vi "SCD - Run Cookbook.vi"(5 "demo":bool, 6 "Timestamp at Start":timestamp=timestamp(3498061709.3036537 s since 1904-01-01), 7 "Neo Info":T10={"Handle"=102, "Pixel Encoding"="Mono16", "AOI Width"=2560, "AOI Height"=2160, "AOI Stride"=5136, "Image Bytes"=11098896, "Image Pixels"=5529600, "Row Readout Time"=9.371428571428572e-06, "Frame Readout Time"=0.010121142857142858, "Interframe Time"=8.434285714285715e-05, "Semaphore"=refnum, "SerialNumber"="SCC-02209", "Camera Model"="DC-152Q-C00-FI", "Controller ID"="3", "Firmware Version"="13.8.26.122", "Shutter"="Global", "Binning"=0, "Time at Synch"=timestamp(3029526000.379448 s since 1904-01-01), "Idx"=0} {"Time at Synch" format="%<%H:%M:%S>T"; "Interframe Time" format="%#_3g"; "Frame Readout Time" format="%_3g"; "Row Readout Time" format="%_3g"}, 8 "Error in":errorcluster, 9 "FITS Header In":T1={"Wavelength (nm)"=530.15, "Exposure (s)"=0.05, "Tuning Delay (ms)"=1000.0, "Beam Type (-1/1)"=1.0, "Tuning Voltages"=[1.111, 2.222, 3.333, 4.444], "Observer"="observer", "Light Shapping Diffuser"=enum."In Beam", "Comment"="", "Data Type"=9, "Mod Cycles"=0, "SCD Calibration Optics"=enum."1 - Polarizer @0, I+Q", "SCD Emission Line Filter"=enum."1-557.6nm", "Cookbook"="", "COMP-S Calibration Wheel"=enum."Dark", "COMP-S Andover Filter Wheel"=enum."530.3nm/HWB 0.34nm (Fe XIV)", "FOV Rotation (deg)"=66.0, "Objective Lens Position (mm)"=0.0, "Occulter size"=0.0, "Time End"=timestamp(3382374145.421875 s since 1904-01-01), "Acc Exposure (s)"=0.0, "Time Stamp Array"=[], "Camera Serial Number"=[], "Camera Temp"=[], "Camera PI (mm)"=[0.0, 0.0, 0.0], "Time Start"=timestamp(3382374145.421875 s since 1904-01-01), "Peripherals"={"ILX controler"=FALSE, "Zone temperatures"=FALSE, "Andor"=FALSE, "Andor 2"=FALSE, "PI Stages"=FALSE, "AISAS mechanisms"=FALSE, "AISAS Mech.lvclass"=refnum, "Zone temp ref"=variant, "FWs"=FALSE}, "FITS paths"=[path " ", path " ", path " ", path " "], "Cameras"=enum."Andor", "load preset cbk"=FALSE, "periodic check count"=0} {"Camera PI (mm)" format="%_3g"; "Acc Exposure (s)" format="%^.3g"; "Occulter size" format="%.2f"; "Objective Lens Position (mm)" min=70.0 max=152.0 format="%.2f"; "FOV Rotation (deg)" format="%.1f"; "Data Type" items=["LIVE", "DARK", "FLAT", "CALI", "OBSE", "ABSO", "AURE", "TARG", "OBJE", "HOLE", "OREX", "THRO", "CHIP"]; "Exposure (s)" format="%^.3g"; "Wavelength (nm)" format="%_6g"}, 10 "FPS":dbl=20.0 format="%0.2p", 11 "Cookbook":T12(array[cluster])=[{"Data Type"=enum."SET EXPOSURE", "Arg 1"=0.1, "Arg 2"=999.0, "Arg 3"=path "C:/SCD Cookbooks/exposure-100ms.rcp", "Comments"=""}, {"Data Type"=enum."ACQUIRE DATA", "Arg 1"=1.0, "Arg 2"=1.0, "Arg 3"=path "C:/SCD Cookbooks/aaa.rcp", "Comments"=""}]) -> (0 "Error out":errorcluster={"status"=FALSE, "code"=5000, "source"="AT Clear All Buffers A.vi\n\nSUCCESS"}, 1 "Headers Out":T1[](array[typedef]) {"Camera PI (mm)" format="%_3g"; "Acc Exposure (s)" format="%^.3g"; "Occulter size" format="%.2f"; "Objective Lens Position (mm)" min=70.0 max=152.0 format="%.2f"; "FOV Rotation (deg)" format="%.1f"; "Data Type" items=["LIVE", "DARK", "FLAT", "CALI", "OBSE", "ABSO", "AURE", "TARG", "OBJE", "HOLE", "OREX", "THRO", "CHIP"]; "Exposure (s)" format="%^.3g"; "Wavelength (nm)" format="%_6g"}, 2 "FITS Path Out":path, 3 "Result":string)   [LabVIEW 2014]
doc: "Use this template to build a VI to use as a subVI."
uses:
  AISAS/Controls/Diffuser.ctl
  <vilib>/Utility/file.llb/Read From Spreadsheet File (DBL).vi
  Controls/SCD - Calibration Optics Filter Wheel.ctl
  Controls/SCD - FITS Cluster.ctl
  Camera/Andor Neo Info.ctl
  Controls/SCD - EDT - Emission Line Filter Wheel.ctl
  Controls/CoMP-S Controls/Polarization Optics Filter Wheel.ctl
  Controls/CoMP-S Controls/Emission Line Filter Wheel.ctl
  AISAS/Controls/focus.ctl
  AISAS/Mech/AISAS Mech.lvclass
  Controls/peripherals.ctl
  Controls/Cameras select.ctl
panel:
  in  "Stop Cookbook":bool
  out "Recipe Being Processed":string
  out "Most Recent Image Accumulation (Modulation State A)":u32[][](graph)
  out "Changes 0 or 1 to true/false for absolute or relative control":bool[](array[boolean])
  out "Updated Header":T1={"Wavelength (nm)"=530.15, "Exposure (s)"=0.05, "Tuning Delay (ms)"=1000.0, "Beam Type (-1/1)"=1.0, "Tuning Voltages"=[1.111, 2.222, 3.333, 4.444], "Observer"="observer", "Light Shapping Diffuser"=enum."In Beam", "Comment"="", "Data Type"=9, "Mod Cycles"=0, "SCD Calibration Optics"=enum."1 - Polarizer @0, I+Q", "SCD Emission Line Filter"=enum."1-557.6nm", "Cookbook"="", "COMP-S Calibration Wheel"=enum."Dark", "COMP-S Andover Filter Wheel"=enum."530.3nm/HWB 0.34nm (Fe XIV)", "FOV Rotation (deg)"=66.0, "Objective Lens Position (mm)"=0.0, "Occulter size"=0.0, "Time End"=timestamp(3382374145.421875 s since 1904-01-01), "Acc Exposure (s)"=0.0, "Time Stamp Array"=[], "Camera Serial Number"=[], "Camera Temp"=[], "Camera PI (mm)"=[0.0, 0.0, 0.0], "Time Start"=timestamp(3382374145.421875 s since 1904-01-01), "Peripherals"={"ILX controler"=FALSE, "Zone temperatures"=FALSE, "Andor"=FALSE, "Andor 2"=FALSE, "PI Stages"=FALSE, "AISAS mechanisms"=FALSE, "AISAS Mech.lvclass"=refnum, "Zone temp ref"=variant, "FWs"=FALSE}, "FITS paths"=[path " ", path " ", path " ", path " "], "Cameras"=enum."Andor", "load preset cbk"=FALSE, "periodic check count"=0} {"Camera PI (mm)" format="%_3g"; "Acc Exposure (s)" format="%^.3g"; "Occulter size" format="%.2f"; "Objective Lens Position (mm)" min=70.0 max=152.0 format="%.2f"; "FOV Rotation (deg)" format="%.1f"; "Data Type" items=["LIVE", "DARK", "FLAT", "CALI", "OBSE", "ABSO", "AURE", "TARG", "OBJE", "HOLE", "OREX", "THRO", "CHIP"]; "Exposure (s)" format="%^.3g"; "Wavelength (nm)" format="%_6g"}
  out "LCVR Voltages":dbl[][](array[numeric])
  out "Total Recipes":i32=2
  out "Recipe Step":i32=1
  out "Mod Cycles":u16=1
  out "Exposure (s)":sgl=0.1
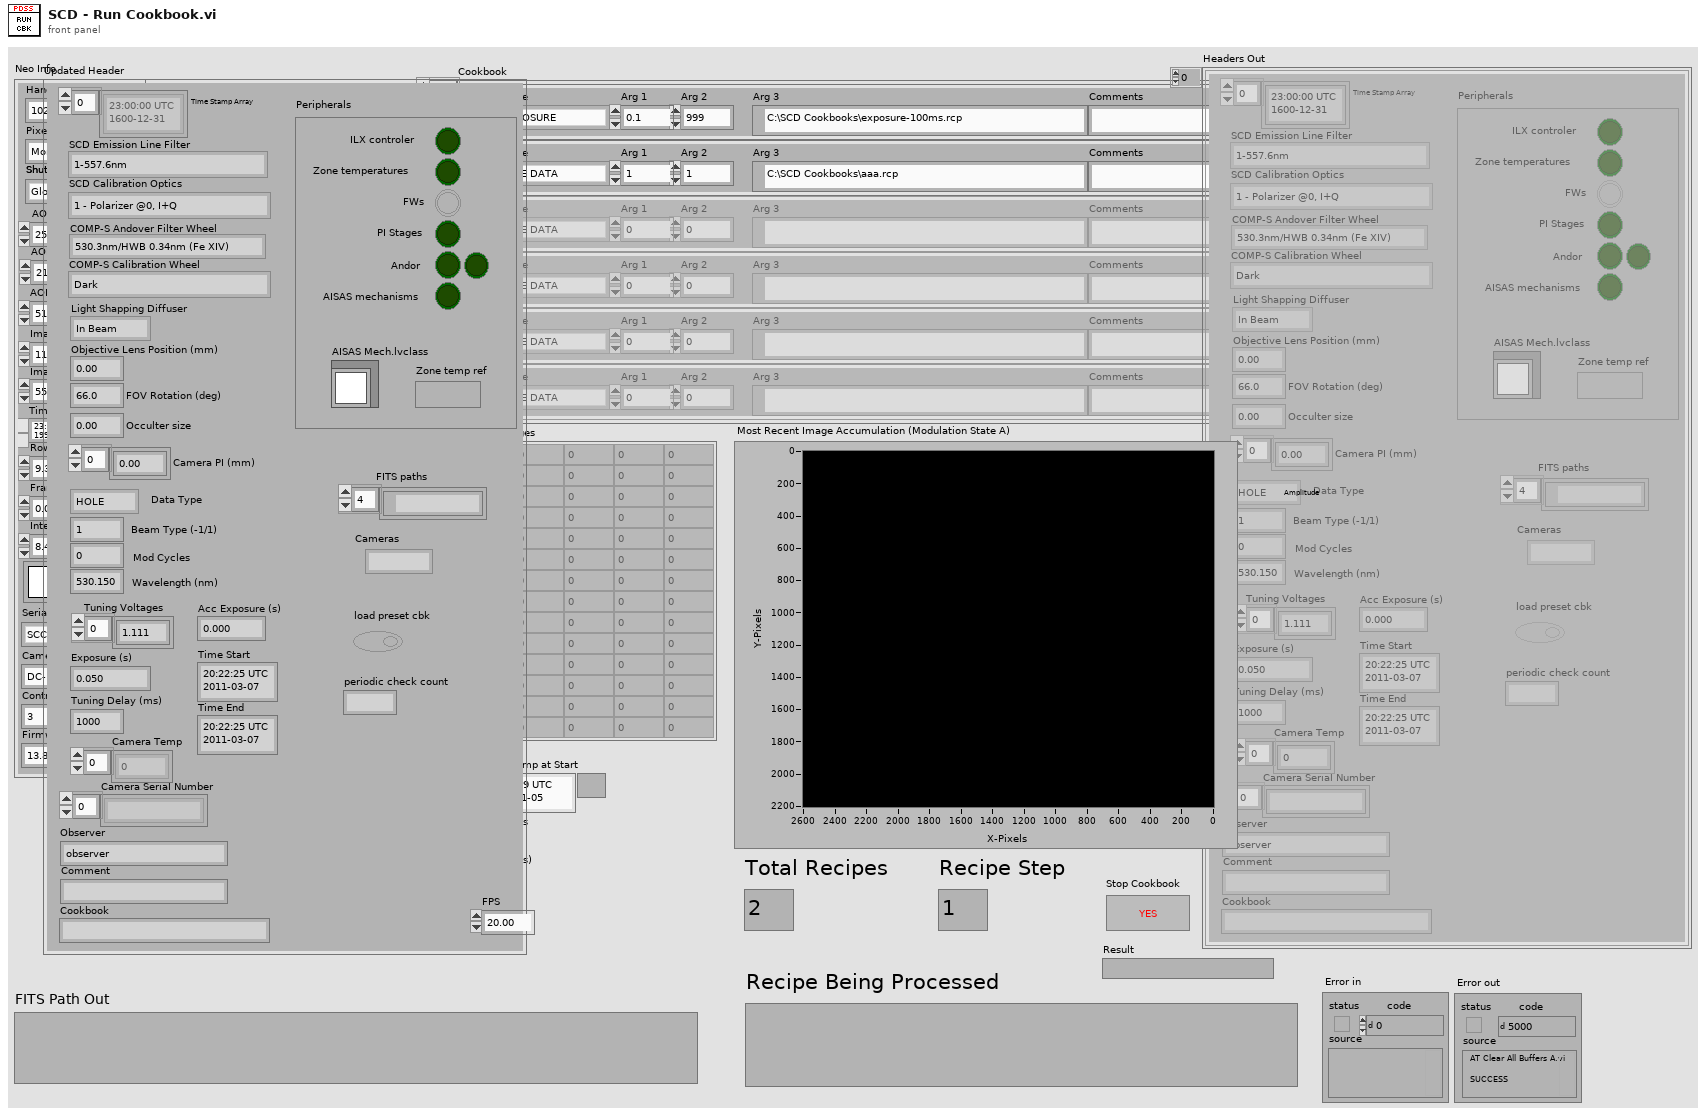
[diagram p1: front panel]
types:
  T1 = typedef "SCD - FITS Cluster.ctl" = cluster{"Wavelength (nm)":dbl, "Exposure (s)":dbl, "Tuning Delay (ms)":dbl, "Beam Type (-1/1)":dbl, "Tuning Voltages":dbl[], "Observer":string, "Light Shapping Diffuser":T2, "Comment":string, "Data Type":u16, "Mod Cycles":u16, "SCD Calibration Optics":T3, "SCD Emission Line Filter":T4, "Cookbook":string, "COMP-S Calibration Wheel":T5, "COMP-S Andover Filter Wheel":T6, "FOV Rotation (deg)":dbl, "Objective Lens Position (mm)":T7, "Occulter size":dbl, "Time End":timestamp, "Acc Exposure (s)":dbl, "Time Stamp Array":timestamp[], "Camera Serial Number":string[], "Camera Temp":dbl[], "Camera PI (mm)":dbl[], "Time Start":timestamp, "Peripherals":T8, "FITS paths":path[], "Cameras":T9, "load preset cbk":bool, "periodic check count":i32}
  T2 = typedef "Diffuser.ctl" = enum16{"Out of Beam", "In Beam"}
  T3 = typedef "SCD - Calibration Optics Filter Wheel.ctl" = enum16{"1 - Polarizer @0, I+Q", "2 - Polarizer @90, I-Q", "3 - Polarizer @45, I+U", "4 - Polarizer @135, I-U", "5 - Polarizer @0, Retarder @45, I+V", "6 - Polarizer @0, Retarder @135, I-V", "7 - Dark", "8 - Clear", "9 - N/A"}
  T4 = typedef "SCD - EDT - Emission Line Filter Wheel.ctl" = enum16{"1-557.6nm", "2-587.6nm", "3-589.6nm", "4-630.2nm", "5-656.4nm", "6-849.8nm", "7-854.2nm", "8-866.2nm", "9-1083.0nm"}
  T5 = typedef "Polarization Optics Filter Wheel.ctl" = enum16{"Dark", "Clear", "Exchange Lens", "Polarizer @0, I+Q", "Polarizer @90, I-Q", "Polarizer @45, I+U", "Polarizer @135, I-U", "Polarizer @0, Retarder @45, I+V", "Polarizer @0, Retarder @135, I-V"}
  T6 = typedef "Emission Line Filter Wheel.ctl" = enum16{"530.3nm/HWB 0.34nm (Fe XIV)", "587.6nm/HBW 0.44nm (He I D3)", "637.5nm/HBW 0.53nm (Fe X)", "656.3nm/HBW 0.57nm (H-Alpha)", "789.2nm/HBW 0.85nm (Fe XI)", "854.2nm/HBW 1.01nm (Ca I)", "1074.7nm/HBW 2.34nm (Fe XIII)", "1079.8nm/HBW 1.64nm (Fe XIII)", "1083.0nm/HBW 1.66nm (He I)"}
  T7 = typedef "focus.ctl" = dbl
  T8 = typedef "peripherals.ctl" = cluster{"ILX controler":bool, "Zone temperatures":bool, "Andor":bool, "Andor 2":bool, "PI Stages":bool, "AISAS mechanisms":bool, "AISAS Mech.lvclass":refnum<class "AISAS Mech.lvclass">, "Zone temp ref":variant, "FWs":bool}
  T9 = typedef "Cameras select.ctl" = enum16{"Andor", "GDR"}
  T10 = typedef "Andor Neo Info.ctl" = cluster{"Handle":i32, "Pixel Encoding":string, "AOI Width":i64, "AOI Height":i64, "AOI Stride":i64, "Image Bytes":i64, "Image Pixels":i64, "Row Readout Time":dbl, "Frame Readout Time":dbl, "Interframe Time":dbl, "Semaphore":T11, "SerialNumber":string, "Camera Model":string, "Controller ID":string, "Firmware Version":string, "Shutter":string, "Binning":u8, "Time at Synch":timestamp, "Idx":i32}
  T11 = typedef "Semaphore RefNum" = refnum<k1>
  T12 = cluster{"Data Type":enum32{"ACQUIRE DATA", "SET DIFFUSER", "CAL-FW", "WAVELENGTH-FW", "INSTR. ROTATION", "MOVE-ABS", "DATATYPE", "SET EXPOSURE", "CBK COMMENTS", "MOVE-REL"}, "Arg 1":sgl, "Arg 2":sgl, "Arg 3":path, "Comments":string}[]
  T13 = enum16{"Emission Line Filters", "Calibration Polarizers"}
  T14 = enum32{"ACQUIRE DATA", "SET DIFFUSER", "CAL-FW", "WAVELENGTH-FW", "INSTR. ROTATION", "MOVE-ABS", "DATATYPE", "SET EXPOSURE", "CBK COMMENTS", "MOVE-REL"}
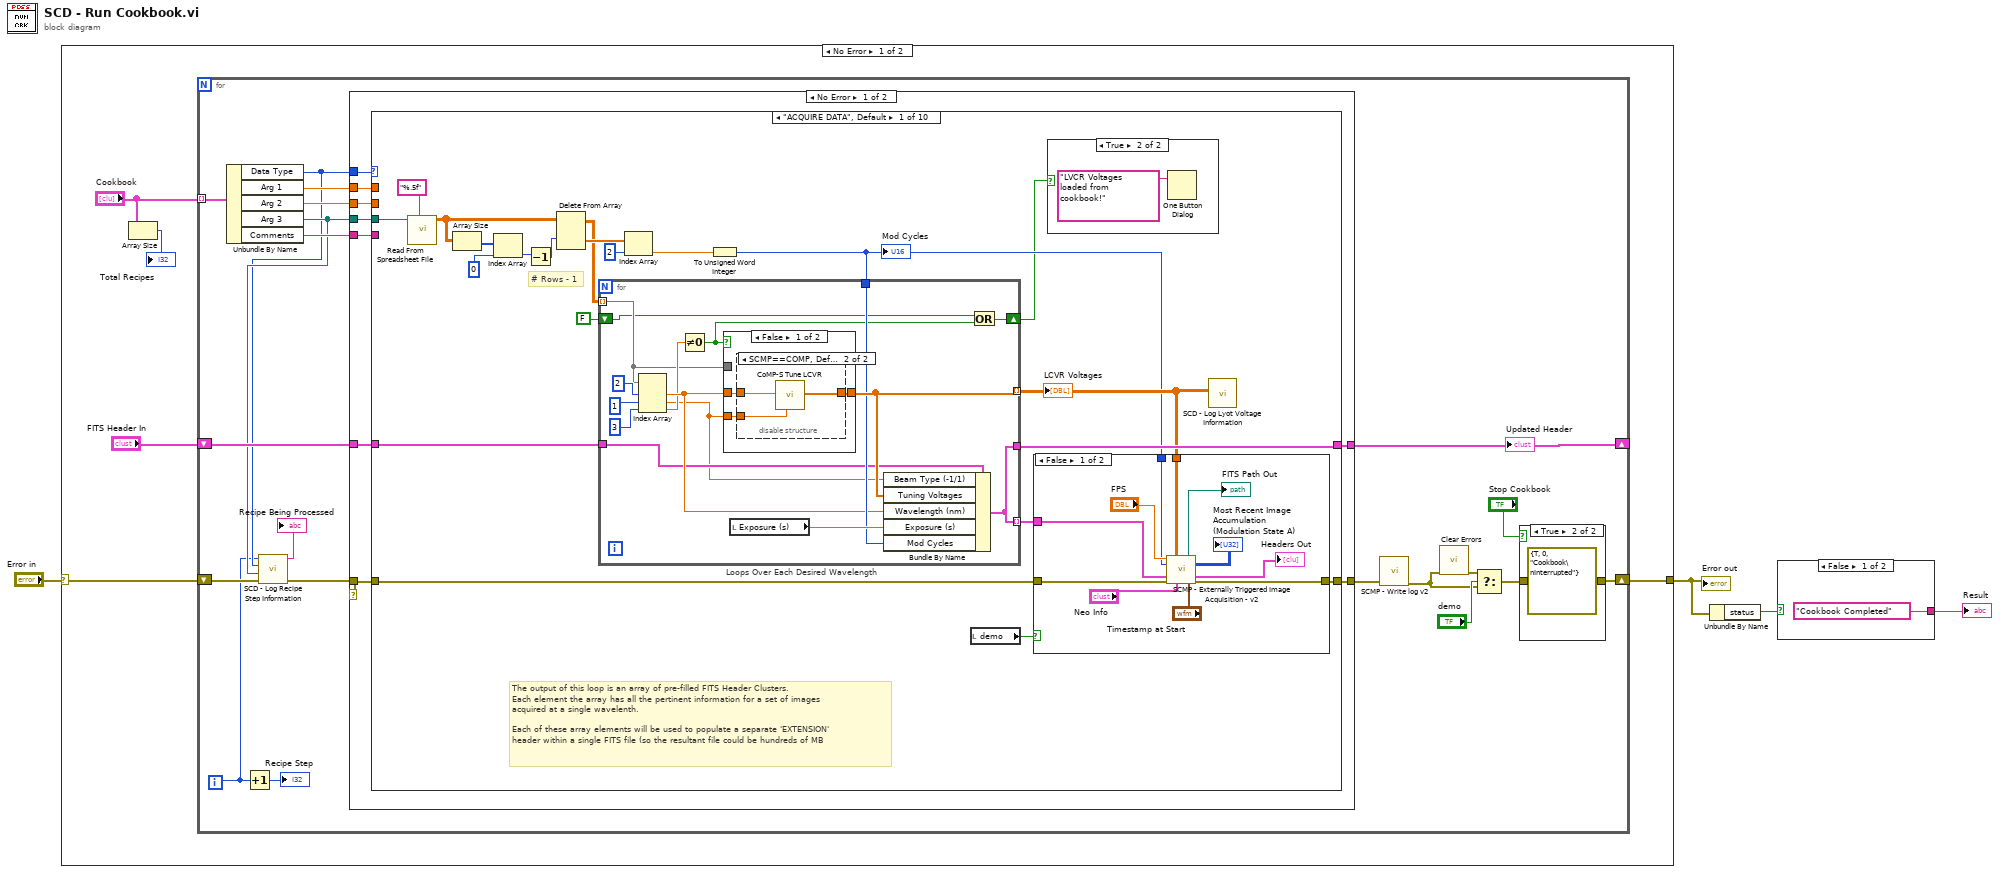
[diagram p0: block diagram]
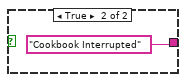
[diagram p2: hidden frame]
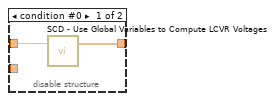
[diagram p6: hidden frame]
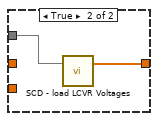
[diagram p7: hidden frame]
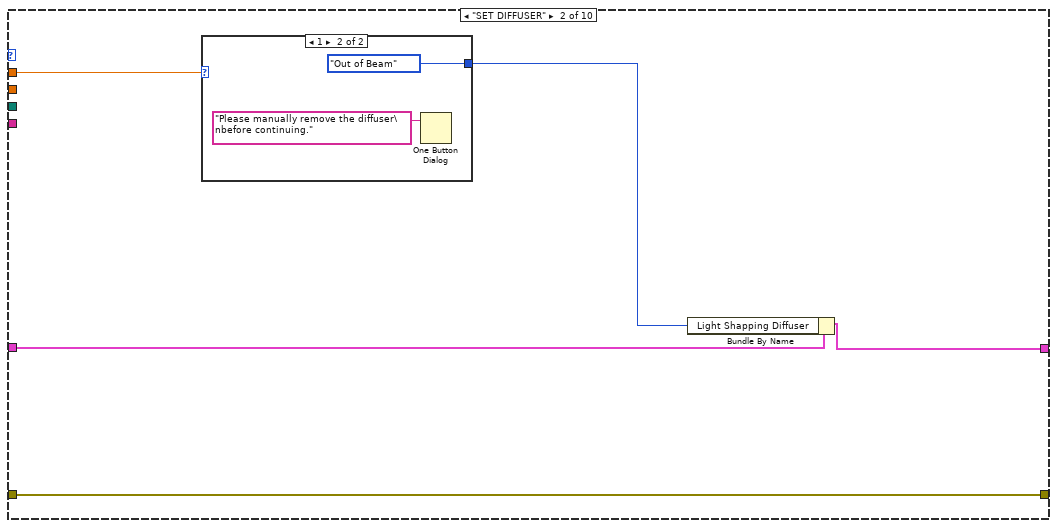
[diagram p8: hidden frame]
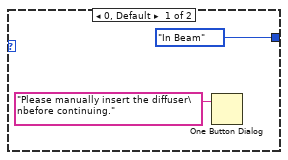
[diagram p9: hidden frame]
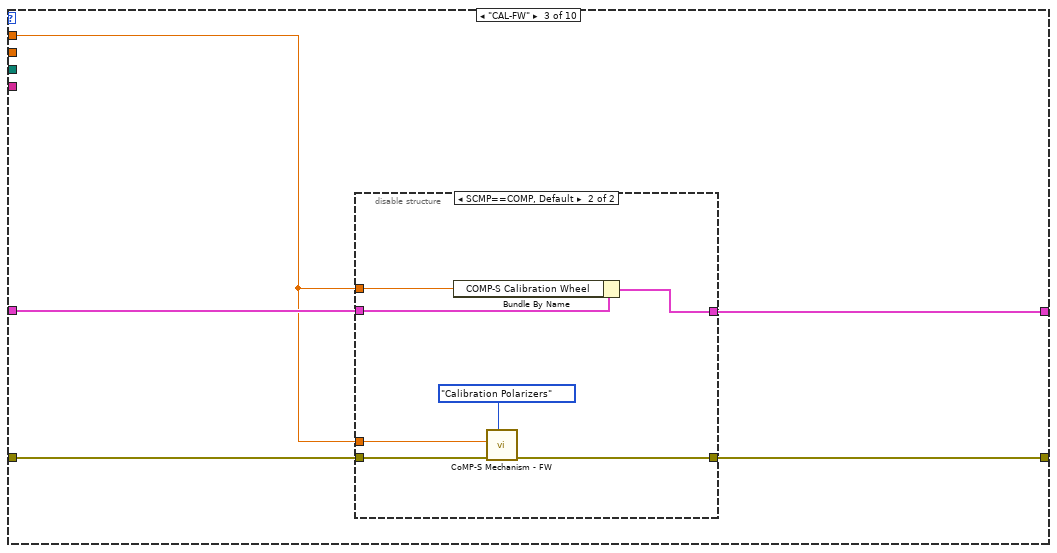
[diagram p10: hidden frame]
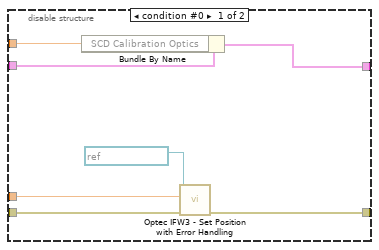
[diagram p11: hidden frame]
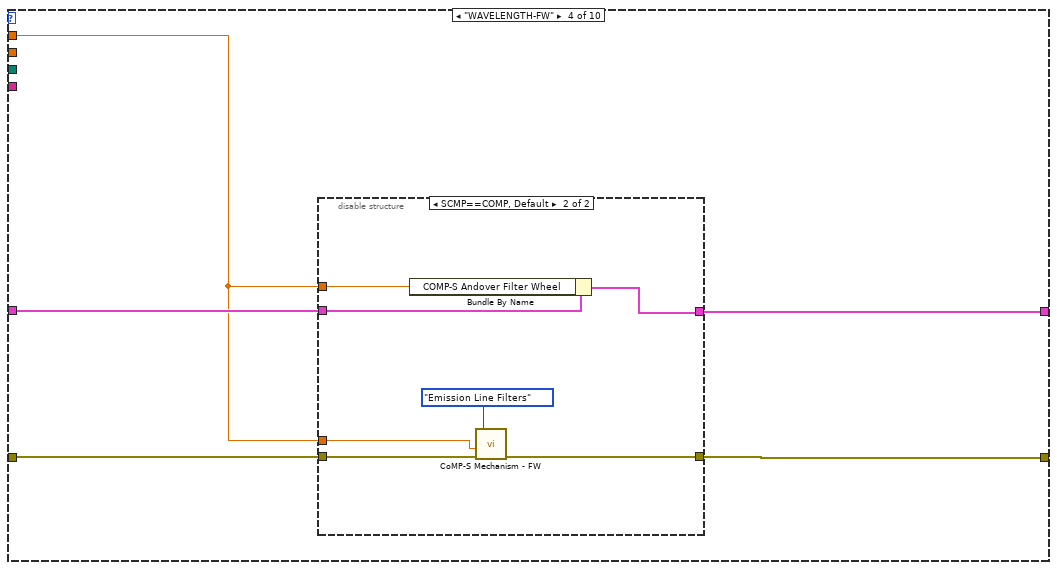
[diagram p12: hidden frame]
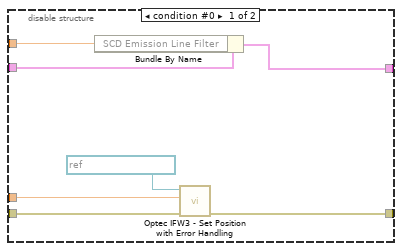
[diagram p13: hidden frame]
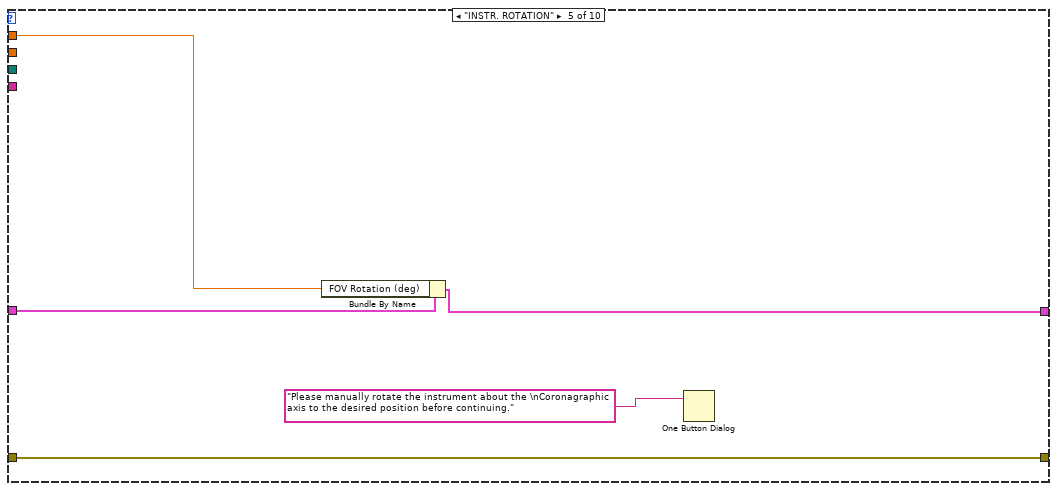
[diagram p14: hidden frame]
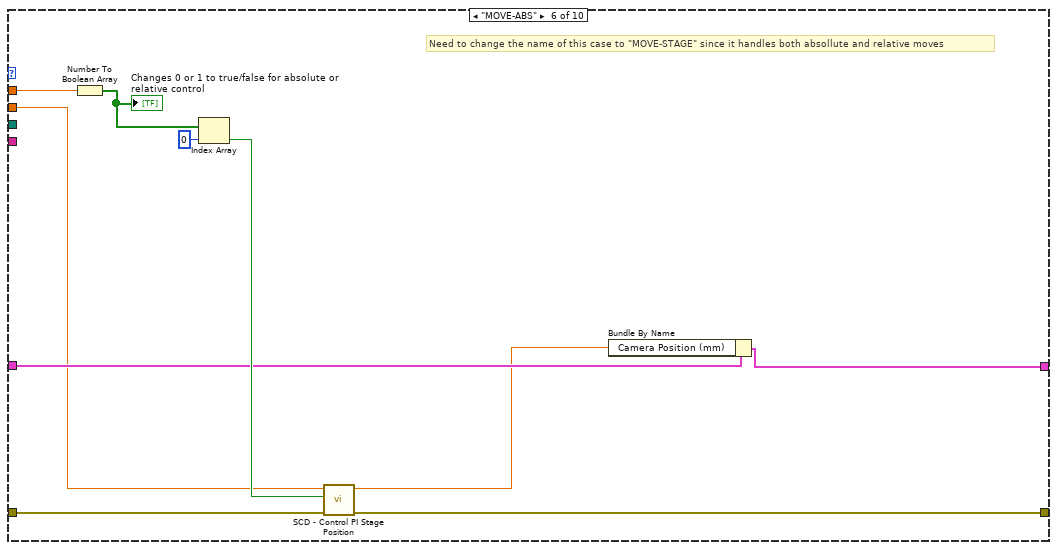
[diagram p15: hidden frame]
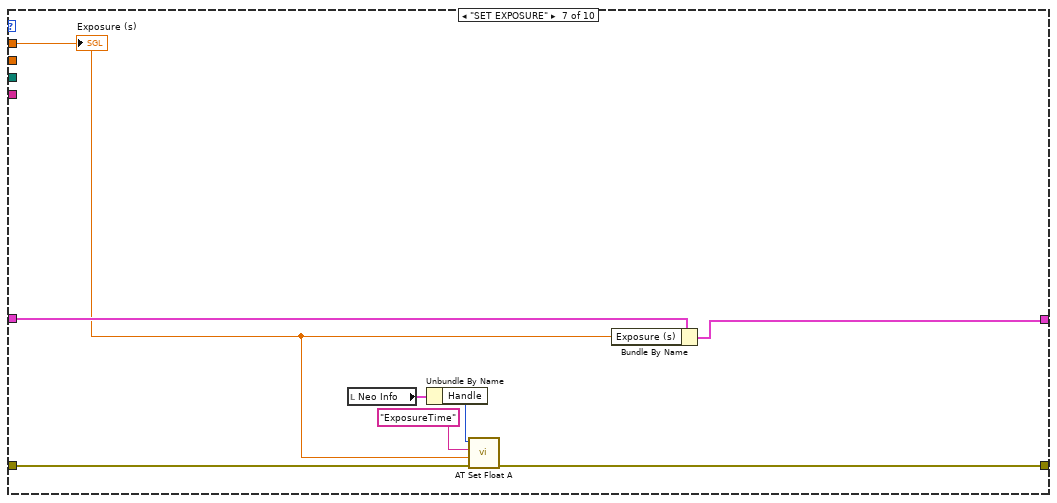
[diagram p16: hidden frame]
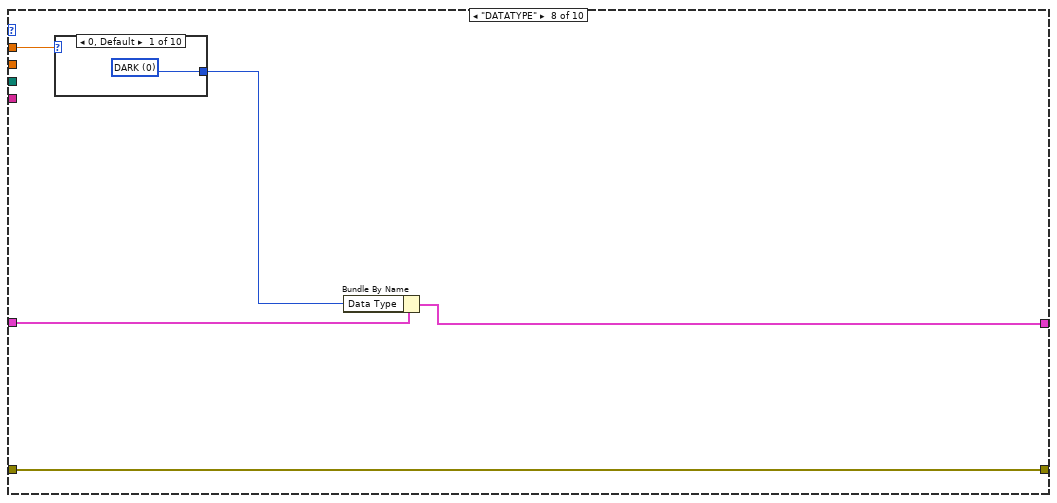
[diagram p17: hidden frame]
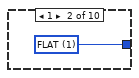
[diagram p18: hidden frame]
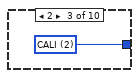
[diagram p19: hidden frame]
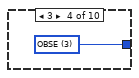
[diagram p20: hidden frame]
diagram:
  n1 = case shown="No Error" "Error in" {
    selector: "Error in" -> [w9 w196]
    tunnel: [w6 w196] -> w3
    frame No Error {
      n2 = Array Size(array="Cookbook") -> (size(s)=→"Total Recipes":i32)
      n3 = for {
        tunnel: "Cookbook" -> [w24] mode=indexing
        shift-right: [w25] -> _
        shift-left: "FITS Header In" -> [w26]
        shift-right: [w20] -> w6
        shift-left: w9 -> [w19]
        i -> [w17]
        n4 = Unbundle By Name(w24) -> ("Data Type"=w18:T14, "Arg 1"=w28:sgl, "Arg 2"=w29:sgl, "Arg 3"=w23:path, "Comments"=w27:string)
        n5 = Increment(x=w17) -> (x+1=→"Recipe Step":i32)
        n6 = call "SCD - Log Recipe Step Information.vi"("error in (no error)"=w19, "Arg 3"=w23, "Data Type"=w18, "Recipe Step"=w17) -> ("error out"=w12:errorcluster, "Recipe Being Processed"=→"Recipe Being Processed":string)  [unwired: 6 in]
        n7 = case shown="No Error" w12 {
          tunnel: w29 -> [w40 _]
          tunnel: w18 -> [w39 _]
          tunnel: w28 -> [w38 _]
          tunnel: w23 -> [w37 _]
          tunnel: w12 -> [w36 w195]
          tunnel: w27 -> [w35 _]
          tunnel: w26 -> [w34 w194]
          tunnel: [w33 w194] -> w25
          tunnel: [w32 w195] -> w11
          frame No Error {
            n8 = case shown="\"ACQUIRE DATA\", Default" w39 {
              tunnel: w40 -> [_ _ _ _ _ w152 _ _ _ _]
              tunnel: w38 -> [_ w101 w109 w128 w149 w159 w166 w171 _ w193]
              tunnel: w37 -> [w61 _ _ _ _ _ _ _ _ _]
              tunnel: w36 -> [w46 w104 w111 w130 w151 w161 w167 w174 w188 w192]
              tunnel: [w50 w104 w110 w129 w151 w160 w165 w174 w187 w191] -> w32
              tunnel: w35 -> [_ _ _ _ _ _ _ _ w186 _]
              tunnel: w34 -> [w52 w103 w112 w132 w150 w155 w169 w173 w185 w189]
              tunnel: [w53 w102 w113 w131 w148 w154 w168 w172 w185 w189] -> w33
              frame "ACQUIRE DATA", Default {
                # "The output of this loop is an array of pre-filled FITS Header Clusters.\nEach element the array has all the pertinent information for a set of images\nacquired at a single wavelenth.\n\nEach of these array elements will be used to populate a separate 'EXTENSION'\nheader within a single FITS file (so the resultant file could be hundreds of MB"
                # "# Rows - 1"
                n9 = call-poly <vilib>:"Read From Spreadsheet File.vi"("format (%.3f)"="%.5f", "file path (dialog if empty)"=w61) -> ("all rows"=w60:dbl[][])  [unwired: 5 in, 4 out]
                n10 = Array Size(array=w60) -> (size(s)=w59:i32[])
                n11 = Index Array(array=w59, index=0) -> (element=w58:i32)
                n12 = Decrement(x=w58) -> (x-1=w57:i32)
                n13 = Delete From Array "Delete From Array"(array=w60, index (row)=w57) -> (deleted portion=w56:dbl[], array with subset deleted=w54:dbl[][])  [unwired: 2 in]
                n14 = Index Array(array=w56, index=2) -> (element=w51:dbl)
                n15 = To Unsigned Word Integer(number=w51) -> (unsigned 16bit integer=w48:u16)
                "Mod Cycles" <- w48
                n16 = for "Loops Over Each Desired Wavelength" {
                  tunnel: w54 -> [w79] mode=indexing
                  tunnel: [w85] -> w49 mode=indexing
                  tunnel: [w86] -> w47 mode=indexing
                  tunnel: w52 -> [w81]
                  tunnel: [w86] -> w53
                  tunnel: w48 -> [w84]
                  shift-right: [w78] -> w42
                  shift-left: FALSE -> [w77]
                  n17 = Index Array(array=w79, index #1=2 ("index"), index #2=1 ("index"), index #3=3 ("index")) -> (element #1=w83:dbl, element #2=w75:dbl, element #3=w80:dbl)
                  n18 = Not Equal To 0?(x=w80) -> (x != 0?=w76:bool)
                  n19 = case shown="False" w76 {
                    tunnel: [w92 w99] -> w85
                    tunnel: w83 -> [w91 _]
                    tunnel: w79 -> [_ w98]
                    tunnel: w75 -> [w90 _]
                    frame False {
                      n20 = disable-structure shown="SCMP==COMP, Default" {
                        disable-tunnel: [w94 w97] -> w92
                        disable-tunnel: w91 -> [w93 w96]
                        disable-tunnel: w90 -> [_ w95]
                        frame condition #0 {
                          n21 = call "SCD - Use Global Variables to Compute LCVR Voltages.vi"("Wavelength (nm)"=w93) -> ("Required LCVR Voltages"=w94:dbl[])  [unwired: 1 in, 1 out]
                        }
                        frame condition #1 (active) {
                          n22 = call "CoMP-S Tune LCVR.vi"("Beam"=w95, "Wavelength (nm)"=w96) -> ("Required LCVR Voltages"=w97:dbl[])  [unwired: 8 in, 1 out]
                        }
                      }
                    }
                    frame True {
                      n23 = call "SCD - load LCVR Voltages.vi"("input rcp"=w98) -> ("Required LCVR Voltages"=w99:dbl[])  [unwired: 2 in]
                    }
                  }
                  n24 = local read "Exposure (s)"() -> (w87:sgl)
                  n25 = Bundle By Name(cluster=w81, "Beam Type (-1/1)"=w75, "Tuning Voltages"=w85, "Wavelength (nm)"=w83, "Exposure (s)"=w87, "Mod Cycles"=w84) -> (w86:T1)
                  n26 = Or(x=w77, y=w76) -> (x .or. y?=w78:bool)
                }
                "LCVR Voltages" <- w49
                n27 = local read "demo"() -> (w43:bool)
                n28 = case shown="False" w43 {
                  tunnel: [w69 w74] -> w50
                  tunnel: w49 -> [w65 _]
                  tunnel: w48 -> [w63 _]
                  tunnel: w47 -> [w72 _]
                  tunnel: w46 -> [w73 w74]
                  frame False {
                    n29 = call "SCMP - Externally Triggered Image Acquisition - v2.vi"("FPS"="FPS", "LCVR Voltages"=w65, "Modulation Cycles"=w63, "Headers In"=w72, "error in"=w73, "Andor Neo"="Neo Info", "Break"="Timestamp at Start") -> ("FITS Path Out"=→"FITS Path Out":path, "Image"=→"Most Recent Image Accumulation (Modulation State A)":u32[][], "Headers Out"=→"Headers Out":T1[], "error out"=w69:errorcluster)  [unwired: 3 in, 2 out]
                  }
                  frame True {
                  }
                }
                n30 = case shown="True" w42 {
                  frame False {
                  }
                  frame True {
                    n31 = One Button Dialog(message="LVCR Voltages loaded from cookbook!") -> ()  [unwired: 1 in, 1 out]
                  }
                }
                n32 = call "SCD - Log Lyot Voltage Information.vi"("array"=w49) -> ()  [unwired: 10 in, 1 out]
              }
              frame "SET DIFFUSER" {
                n33 = case shown="1" w101 {
                  tunnel: [Diffuser."In Beam" ("Light Shapping Diffuser") Diffuser."Out of Beam" ("Light Shapping Diffuser")] -> w100
                  frame 0, Default {
                    n34 = One Button Dialog(message="Please manually insert the diffuser\nbefore continuing.") -> ()  [unwired: 1 in, 1 out]
                  }
                  frame 1 {
                    n35 = One Button Dialog(message="Please manually remove the diffuser\nbefore continuing.") -> ()  [unwired: 1 in, 1 out]
                  }
                }
                n36 = Bundle By Name(cluster=w103, "Light Shapping Diffuser"=w100) -> (w102:T1)
              }
              frame "CAL-FW" {
                n37 = disable-structure shown="SCMP==COMP, Default" {
                  disable-tunnel: [w120 w125] -> w113
                  disable-tunnel: w112 -> [w119 w126]
                  disable-tunnel: w109 -> [w117 w127]
                  disable-tunnel: w111 -> [w116 w124]
                  disable-tunnel: [w115 w123] -> w110
                  disable-tunnel: w109 -> [w114 w121]
                  frame condition #0 {
                    n38 = Bundle By Name(cluster=w119, "SCD Calibration Optics"=w117) -> (w120:T1)
                    n39 = call "Optec IFW3 - Set Position with Error Handling.vi"("error in"=w116, "Emission Line Filter"=w114, "Filter Wheel Selector"=refnum<visa-resource-name> "Cal-Optics" ("Filter Wheel (Andover or Cal Optics)")) -> ("error out"=w115:errorcluster)  [unwired: 6 in, 2 out]
                  }
                  frame condition #1 (active) {
                    n40 = Bundle By Name(cluster=w126, "COMP-S Calibration Wheel"=w127) -> (w125:T1)
                    n41 = call "CoMP-S Mechanism - FW.vi"("error in (no error)"=w124, "Calibration Polarizer Filters [Dark]"=w121, "Filter Wheel Selector"=T13."Calibration Polarizers") -> ("error out"=w123:errorcluster)  [unwired: 5 in, 3 out]
                  }
                }
              }
              frame "WAVELENGTH-FW" {
                n42 = disable-structure shown="SCMP==COMP, Default" {
                  disable-tunnel: w132 -> [w139 w145]
                  disable-tunnel: [w138 w144] -> w131
                  disable-tunnel: w128 -> [w136 w146]
                  disable-tunnel: w130 -> [w135 w143]
                  disable-tunnel: [w134 w142] -> w129
                  disable-tunnel: w128 -> [w133 w140]
                  frame condition #0 {
                    n43 = Bundle By Name(cluster=w139, "SCD Emission Line Filter"=w136) -> (w138:T1)
                    n44 = call "Optec IFW3 - Set Position with Error Handling.vi"("error in"=w135, "Emission Line Filter"=w133, "Filter Wheel Selector"=refnum<visa-resource-name> "Andover-Filters" ("Filter Wheel (Andover or Cal Optics)")) -> ("error out"=w134:errorcluster)  [unwired: 6 in, 2 out]
                  }
                  frame condition #1 (active) {
                    n45 = Bundle By Name(cluster=w145, "COMP-S Andover Filter Wheel"=w146) -> (w144:T1)
                    n46 = call "CoMP-S Mechanism - FW.vi"("error in (no error)"=w143, "Emission Line Filters [530.3 nm]"=w140, "Filter Wheel Selector"=T13."Emission Line Filters") -> ("error out"=w142:errorcluster)  [unwired: 5 in, 3 out]
                  }
                }
              }
              frame "INSTR. ROTATION" {
                n47 = Bundle By Name(cluster=w150, "FOV Rotation (deg)"=w149) -> (w148:T1)
                n48 = One Button Dialog(message="Please manually rotate the instrument about the \nCoronagraphic axis to the desired position before continuing.") -> ()  [unwired: 1 in, 1 out]
              }
              frame "MOVE-ABS" {
                # "Need to change the name of this case to \"MOVE-STAGE\" since it handles both absollute and relative moves"
                n49 = Number To Boolean Array(number=w159) -> (Boolean array=w158:bool[])
                "Changes 0 or 1 to true/false for absolute or relative control" <- w158
                n50 = Index Array(array=w158, index=0) -> (element=w156:bool)
                n51 = call "SCD - Control PI Stage Position.vi"("error in"=w161, "Absolute (F) or \nRelative (T) Move"=w156, "Desired Camera Move"=w152) -> ("error out"=w160:errorcluster, "Camera Finish Position"=w153:dbl)  [unwired: 7 in]
                n52 = Bundle By Name(cluster=w155, "Camera Position (mm)"=w153) -> (w154:T1)
              }
              frame "SET EXPOSURE" {
                n53 = local read "Neo Info"() -> (w164:T10)
                n54 = Unbundle By Name(w164) -> ("Handle"=w163:i32)
                n55 = call <userlib>:"AT Set Float A.vi"("error in (no error)"=w167, "Value"=w166, "Feature"="ExposureTime", "Hndl"=w163) -> ("error out"=w165:errorcluster)  [unwired: 6 in, 1 out]
                n56 = Bundle By Name(cluster=w169, "Exposure (s)"=w166) -> (w168:T1)
                "Exposure (s)" <- w166
              }
              frame "DATATYPE" {
                n57 = case shown="0, Default" w171 {
                  tunnel: [w175 w176 w177 w178 w179 w180 w181 w182 w183 w184] -> w170
                  frame 0, Default {
                    w175 = u16 0 items=["DARK", "FLAT", "CALI", "OBSE", "ABSO", "AURE", "TARG", "OBJE", "HOLE", "LIVE"] ("Data Type")
                  }
                  frame 1 {
                    w176 = u16 1 items=["DARK", "FLAT", "CALI", "OBSE", "ABSO", "AURE", "TARG", "OBJE", "HOLE", "LIVE"] ("Data Type")
                  }
                  frame 2 {
                    w177 = u16 2 items=["DARK", "FLAT", "CALI", "OBSE", "ABSO", "AURE", "TARG", "OBJE", "HOLE", "LIVE"] ("Data Type")
                  }
                  frame 3 {
                    w178 = u16 3 items=["DARK", "FLAT", "CALI", "OBSE", "ABSO", "AURE", "TARG", "OBJE", "HOLE", "LIVE"] ("Data Type")
                  }
                  frame 4 {
                    w179 = u16 4 items=["DARK", "FLAT", "CALI", "OBSE", "ABSO", "AURE", "TARG", "OBJE", "HOLE", "LIVE"] ("Data Type")
                  }
                  frame 5 {
                    w180 = u16 5 items=["DARK", "FLAT", "CALI", "OBSE", "ABSO", "AURE", "TARG", "OBJE", "HOLE", "LIVE"] ("Data Type")
                  }
                  frame 6 {
                    w181 = u16 6 items=["DARK", "FLAT", "CALI", "OBSE", "ABSO", "AURE", "TARG", "OBJE", "HOLE", "LIVE"] ("Data Type")
                  }
                  frame 7 {
                    w182 = u16 7 items=["DARK", "FLAT", "CALI", "OBSE", "ABSO", "AURE", "TARG", "OBJE", "HOLE", "LIVE"] ("Data Type")
                  }
                  frame 8 {
                    w183 = u16 8 items=["DARK", "FLAT", "CALI", "OBSE", "ABSO", "AURE", "TARG", "OBJE", "HOLE", "LIVE"] ("Data Type")
                  }
                  frame 9 {
                    w184 = u16 9 items=["DARK", "FLAT", "CALI", "OBSE", "ABSO", "AURE", "TARG", "OBJE", "HOLE", "LIVE"] ("Data Type")
                  }
                }
                n58 = Bundle By Name(cluster=w173, "Data Type"=w170) -> (w172:T1)
              }
              frame "CBK COMMENTS" {
                n59 = call "SCMP - Write log v2.vi"("Error to log"=w188, "data"=w186) -> ("error out"=w187:errorcluster)  [unwired: 7 in, 2 out]
              }
              frame "MOVE-REL" {
                w190 = TRUE  # Relative Move
                n60 = call "SCD - Control PI Stage Position.vi"("error in"=w192, "Absolute (F) or \nRelative (T) Move"=w190, "Desired Camera Move"=w193) -> ("error out"=w191:errorcluster)  [unwired: 7 in, 1 out]
              }
            }
          }
          frame Error {
          }
        }
        "Updated Header" <- w25
        n61 = call "SCMP - Write log v2.vi"("Error to log"=w11) -> ("error out"=w10:errorcluster)  [unwired: 8 in, 2 out]
        n62 = call <vilib>:"Clear Errors.vi"("error in (no error)"=w10) -> ("error out"=w16:errorcluster)  [unwired: 5 in, 1 out]
        n63 = Select(t=w16, s="demo", f=w10) -> (s? t:f=w14:errorcluster)
        n64 = case shown="True" "Stop Cookbook" {
          tunnel: w14 -> [w30 _]
          tunnel: [w30 errorcluster {"status"=TRUE, "code"=0, "source"="Cookbook\nInterrupted"} ("error IO")] -> w20
          frame False {
          }
          frame True {
          }
        }
      }
    }
    frame Error {
    }
  }
  "Error out" <- w3
  n65 = Unbundle By Name(w3) -> ("status"=w2:bool)
  n66 = case shown="False" w2 {
    tunnel: ["Cookbook Completed" ("data") "Cookbook Interrupted" ("data")] -> w1
    frame False {
    }
    frame True {
    }
  }
  "Result" <- w1
